vi "wd_length_append.vi"(8 "error in (no error)":errorcluster, 9 "channel index (0)":u32, 10 "data size":u64, 11 "meta in":T1={"TargetFile"=path "", "StreamMode"=enum."File", "Append?"=FALSE, "ChunkSize"=0, "TimeColumnMode"=enum."Empty", "TimestampFormat"="", "AbsoluteTime?"=FALSE, "FileAttribute "={"Creator"="", "Title"="", "SheetName"=""}, "Column"=[], "FileRef"=refnum, "MemoryRef"=[], "RecordInfo"=[], " ChannelPreviousInfo"=[], "ChannelFirstRecord"=[], "PredefinedFormattedValueLength"=20, "DiskTemplate"={"XMLRef"=[refnum, refnum, refnum, refnum, refnum, refnum], "ZipPath"=path "", "MetaFile"={"Ref"=refnum, "NextRow"=0, "NextPosition"=0, "Block"=[]}, "TempFolder"=path ""}}) -> (0 "error out":errorcluster, 3 "meta out":T1={"TargetFile"=path "", "StreamMode"=enum."File", "Append?"=FALSE, "ChunkSize"=0, "TimeColumnMode"=enum."Empty", "TimestampFormat"="", "AbsoluteTime?"=FALSE, "FileAttribute "={"Creator"="", "Title"="", "SheetName"=""}, "Column"=[], "FileRef"=refnum, "MemoryRef"=[], "RecordInfo"=[], " ChannelPreviousInfo"=[], "ChannelFirstRecord"=[], "PredefinedFormattedValueLength"=20, "DiskTemplate"={"XMLRef"=[refnum, refnum, refnum, refnum, refnum, refnum], "ZipPath"=path "", "MetaFile"={"Ref"=refnum, "NextRow"=0, "NextPosition"=0, "Block"=[]}, "TempFolder"=path ""}})   [LabVIEW 2020, in "NI_ExcelFile.lvlib"]
uses:
  <vilib>/express/express shared/NI_ExcelFile/NI_ExcelFile.lvlib
  <vilib>/express/express shared/NI_ExcelFile/Ctrls/MainData.ctl
  <vilib>/express/express shared/NI_ExcelFile/Ctrls/StreamMode.ctl
  <vilib>/express/express shared/NI_ExcelFile/Ctrls/TimeColumnMode.ctl
  <vilib>/express/express shared/NI_ExcelFile/Ctrls/FileAttribute.ctl
  <vilib>/express/express shared/NI_ExcelFile/Ctrls/Columns.ctl
  <vilib>/express/express shared/NI_ExcelFile/Ctrls/ColumnInfo.ctl
  <vilib>/express/express shared/NI_ExcelFile/Ctrls/DataType.ctl
  <vilib>/express/express shared/NI_ExcelFile/Ctrls/wd_recordInfo.ctl
  <vilib>/express/express shared/NI_ExcelFile/Ctrls/disk_TemplateFile.ctl
  <vilib>/express/express shared/NI_ExcelFile/Ctrls/meta_file.ctl
  <vilib>/express/express shared/NI_ExcelFile/Ctrls/meta_Block.ctl
  <vilib>/express/express shared/NI_ExcelFile/Ctrls/meta_BlockType.ctl
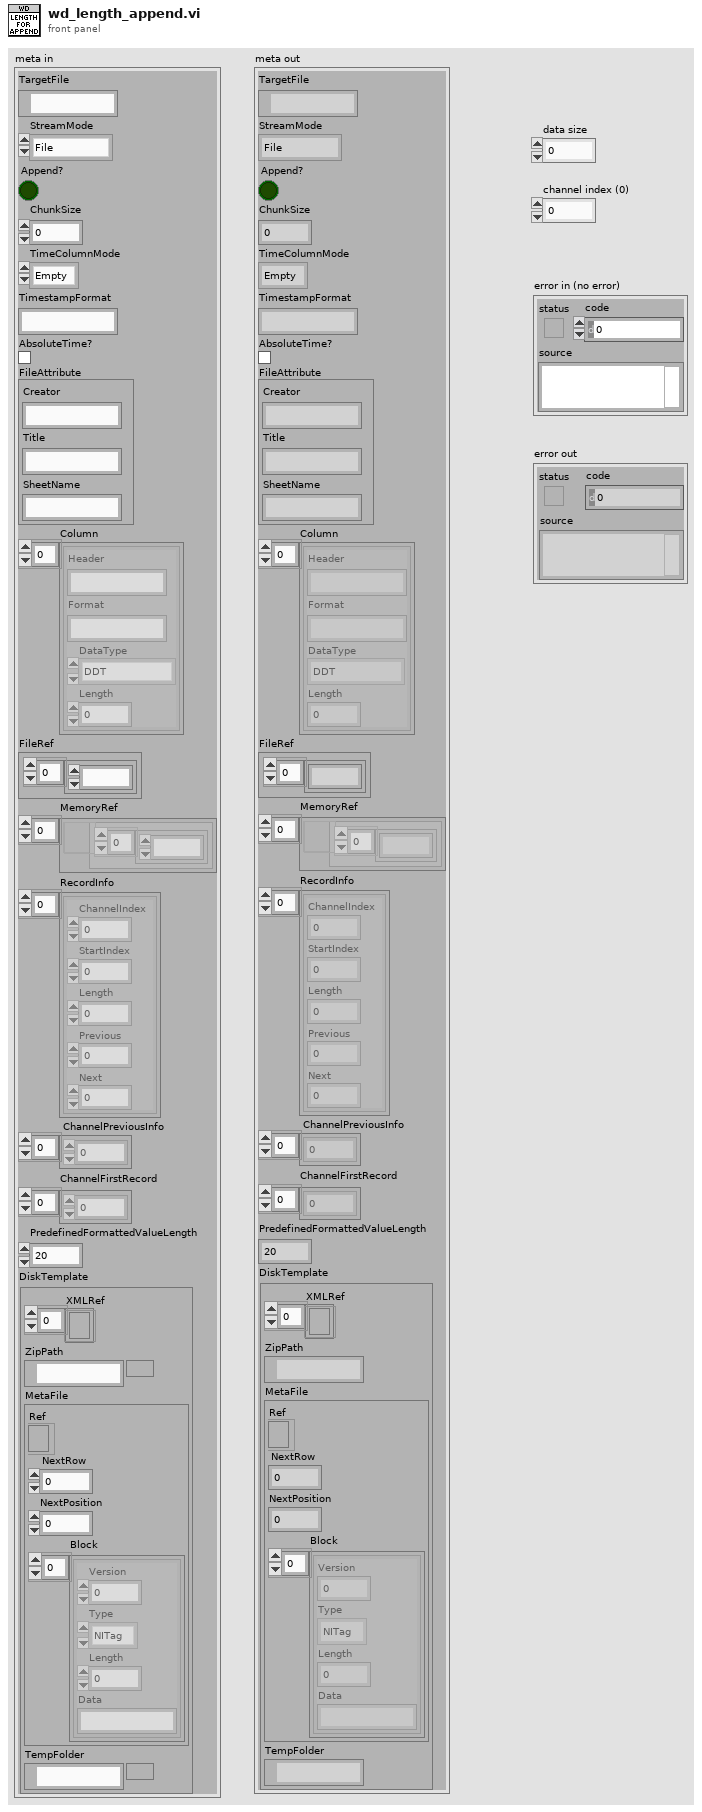
[diagram p1: front panel]
types:
  T1 = typedef "NI_ExcelFile.lvlib/MainData.ctl" = cluster{"TargetFile":path, "StreamMode":T2, "Append?":bool, "ChunkSize":u64, "TimeColumnMode":T3, "TimestampFormat":string, "AbsoluteTime?":bool, "FileAttribute ":T4, "Column":T5, "FileRef":refnum<k1>, "MemoryRef":refnum<data-value>[], "RecordInfo":T8[], " ChannelPreviousInfo":u32[], "ChannelFirstRecord":u32[], "PredefinedFormattedValueLength":i64, "DiskTemplate":T9}
  T2 = typedef "NI_ExcelFile.lvlib/StreamMode.ctl" = enum16{"File", "Memory"}
  T3 = typedef "NI_ExcelFile.lvlib/TimeColumnMode.ctl" = enum16{"Empty", "OnePerCh", "One"}
  T4 = typedef "NI_ExcelFile.lvlib/FileAttribute.ctl" = cluster{"Creator":string, "Title":string, "SheetName":string}
  T5 = typedef "NI_ExcelFile.lvlib/Columns.ctl" = T6[]
  T6 = typedef "NI_ExcelFile.lvlib/ColumnInfo.ctl" = cluster{"Header":string, "Format":string, "DataType":T7, "Length":u64}
  T7 = typedef "NI_ExcelFile.lvlib/DataType.ctl" = enum16{"DDT", "WFM", "Array of STR", "Array of DBL", "Array of I8", "Array of I16", "Array of I32", "Array of I64", "Array of SGL", "Array of U8", "Array of U16", "Array of U32", "Array of U64", "Array of Time"}
  T8 = typedef "NI_ExcelFile.lvlib/wd_recordInfo.ctl" = cluster{"ChannelIndex":u32, "StartIndex":u64, "Length":u64, "Previous":i32, "Next":i32}
  T9 = typedef "NI_ExcelFile.lvlib/disk_TemplateFile.ctl" = cluster{"XMLRef":refnum<file>[], "ZipPath":path, "MetaFile":T10, "TempFolder":path}
  T10 = typedef "NI_ExcelFile.lvlib/meta_file.ctl" = cluster{"Ref":refnum<file>, "NextRow":i32, "NextPosition":i64, "Block":T11[]}
  T11 = typedef "NI_ExcelFile.lvlib/meta_Block.ctl" = cluster{"Version":u16, "Type":T12, "Length":i32, "Data":string}
  T12 = typedef "NI_ExcelFile.lvlib/meta_BlockType.ctl" = enum16{"NITag", "File", "Column"}
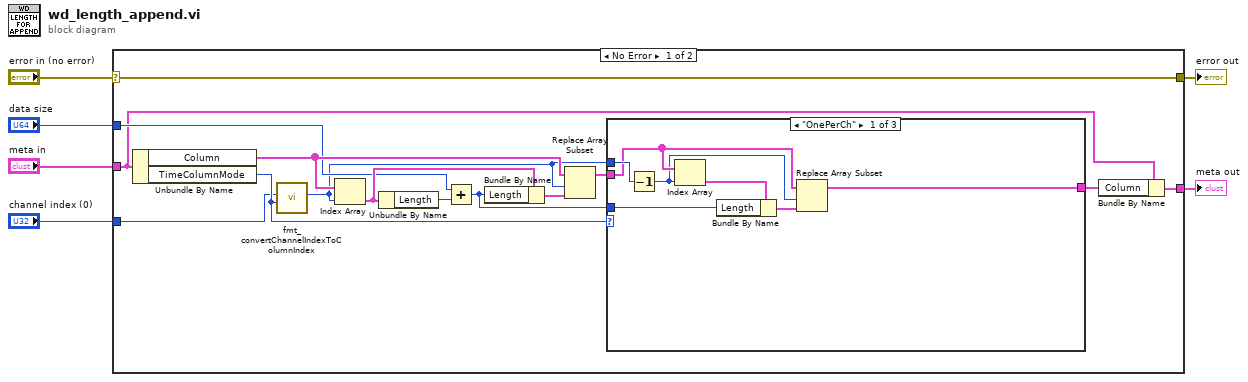
[diagram p0: block diagram]
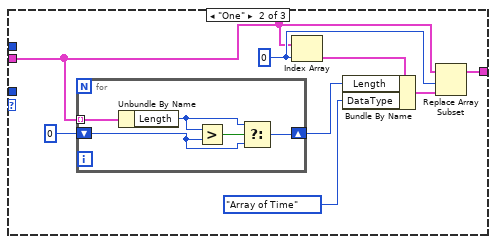
[diagram p2: hidden frame]
diagram:
  n1 = case shown="No Error" "error in (no error)" {
    selector: "error in (no error)" -> [w8 w42]
    tunnel: "meta in" -> [w7 w43]
    tunnel: "channel index (0)" -> [w10 _]
    tunnel: [w15 w43] -> w4
    tunnel: [w8 w42] -> w2
    tunnel: "data size" -> [w12 _]
    frame No Error {
      n2 = Unbundle By Name(w7) -> ("Column"=w20:T5, "TimeColumnMode"=w11:T3)
      n3 = call <vilib>:"fmt_convertChannelIndexToColumnIndex.vi"("TimeColumnMode"=w11, "channel index"=w10) -> ("data column index"=w9:i32)  [unwired: 8 in, 1 out]
      n4 = Index Array(array=w20, index=w9) -> (element=w19:T6)
      n5 = Unbundle By Name(w19) -> ("Length"=w18:u64)
      n6 = Add(x=w12, y=w18) -> (x+y=w17:u64)
      n7 = Bundle By Name(cluster=w19, "Length"=w17) -> (w14:T6)
      n8 = Replace Array Subset(array=w20, new element=w14, index=w9) -> (w13:T5)
      n9 = case shown="\"OnePerCh\"" w11 {
        tunnel: [w21 w34 w41] -> w16
        tunnel: w13 -> [w24 w28 w41]
        tunnel: w9 -> [w27 _ _]
        tunnel: w17 -> [w25 _ _]
        frame "OnePerCh" {
          n10 = Decrement(x=w27) -> (x-1=w22:i32)
          n11 = Index Array(array=w24, index=w22) -> (element=w26:T6)
          n12 = Bundle By Name(cluster=w26, "Length"=w25) -> (w23:T6)
          n13 = Replace Array Subset(array=w24, new element=w23, index=w22) -> (w21:T5)
        }
        frame "One" {
          w29 = 0 ("index")
          n14 = for {
            tunnel: w28 -> [w40] mode=indexing
            shift-right: [w37] -> w33
            shift-left: u64 0 -> [w38]
            n15 = Unbundle By Name(w40) -> ("Length"=w36:u64)
            n16 = Greater?(x=w36, y=w38) -> (0:w39:bool)
            n17 = Select(t=w36, s=w39, f=w38) -> (s? t:f=w37:u64)
          }
          n18 = Index Array(array=w28, index=w29) -> (element=w30:T6)
          n19 = Bundle By Name(cluster=w30, "Length"=w33, "DataType"=DataType."Array of Time" ("Column DataType")) -> (w31:T6)
          n20 = Replace Array Subset(array=w28, new element=w31, index=w29) -> (w34:T5)
        }
        frame "Empty", Default {
        }
      }
      n21 = Bundle By Name(cluster=w7, "Column"=w16) -> (w15:T1)
    }
    frame Error {
    }
  }
  "meta out" <- w4
  "error out" <- w2
